vi "to string.vi"(8 "error in":errorcluster, 11 "Engine configuration in":refnum<class "Engine configuration.lvclass">) -> (0 "error out":errorcluster, 1 "data":string, 2 "version":string, 3 "Engine configuration out":refnum<class "Engine configuration.lvclass">)   [LabVIEW 2025, in "Abstract Engine.lvlib" / "Engine configuration.lvclass"]
doc: "Provides an interface for saving a module configuration to a file or other serialized data source. It is recommended that all children of this class store data in two sets--data required for its own initialization, and any data required for parent initialization--and that each implementation uses the <b>Call Parent Method</b> primitive to serialize parent information.Copyright 2017 National Instruments Corporation\n\nLicensed under the Apache License, Version 2.0 (the \"License\"); you may not use this file except in compliance with the License. You may obtain a copy of the License at http://www.apache.org/licenses/LICENSE-2.0\nUnless required by applicable law or agreed to in writing, software distributed under the License is distributed on an \"AS IS\" BASIS, WITHOUT WARRANTIES OR CONDITIONS OF ANY KIND, either express or implied. See the License for the specific language governing permissions and limitations under the License."
uses:
  Engine configuration.lvclass
  Engine configuration.lvclass/Engine configuration.ctl
  Users/Public/Documents/Sandia National Labs/TSS Plugin/CEF.lvlibp/serializable configuration/CEF_serializable configuration.lvclass
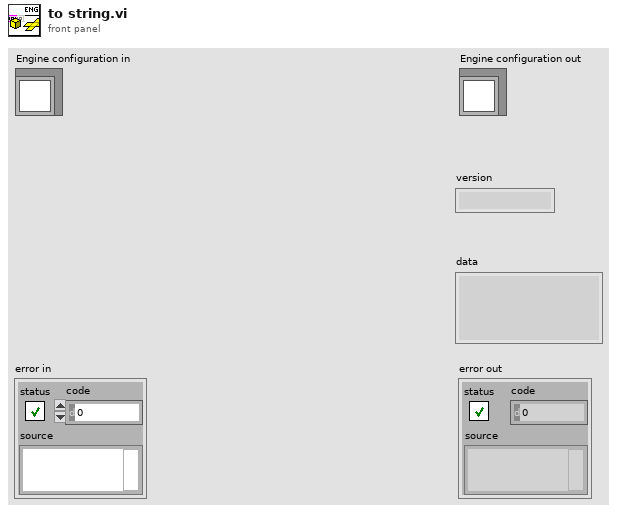
[diagram p1: front panel]
types:
  T1 = typedef "Abstract Engine.lvlib/Engine configuration.lvclass/Engine Setting.ctl" = cluster{"Enabled":bool, "IP Address":string, "Port":i32, "Initialize Order":i32, "Description":string, "Version":string, "Type":string}
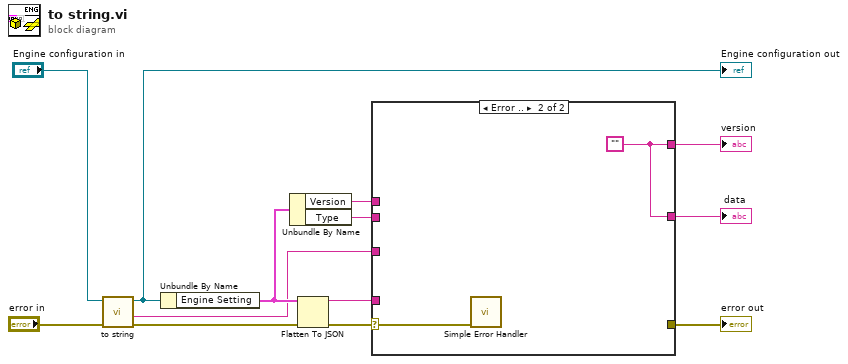
[diagram p0: block diagram]
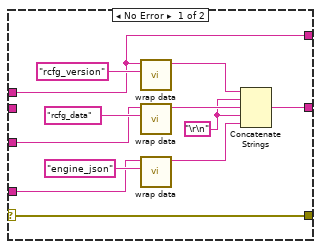
[diagram p2: hidden frame]
diagram:
  n1 = call-parent "to string.vi"("error in"="error in", "CEF_Configuration in"="Engine configuration in") -> ("error out"=w10:errorcluster, "data"=w4:string, "CEF_Configuration out"=w11:refnum<class "Engine configuration.lvclass">)  [unwired: 6 in, 1 out]
  "Engine configuration out" <- w11
  n2 = Unbundle By Name(w11) -> ("Engine Setting"=w9:T1)
  n3 = Unbundle By Name(w9) -> ("Version"=w3:string, "Type"=w1:string)
  n4 = Flatten To JSON(anything=w9, error in (no error)=w10) -> (JSON string=w7:string, 11:w8:errorcluster)  [unwired: 1 in]
  n5 = case shown="Error .." w8 {
    selector: w8 -> [w25 w26]
    tunnel: [w25 _] -> w5
    tunnel: w7 -> [w21 _]
    tunnel: w4 -> [w19 _]
    tunnel: [w18 w27] -> w6
    tunnel: w3 -> [w14 _]
    tunnel: [w14 w27] -> w2
    tunnel: w1 -> [_ _]
    frame No Error {
      w16 = "\r\n"
      n6 = call "wrap data.vi"("identifier"="rcfg_version" ("additional identifier"), "data to wrap"=w14) -> ("wrapped data"=w15:string)  [unwired: 9 in]
      n7 = call "wrap data.vi"("identifier"="rcfg_data" ("additional identifier"), "data to wrap"=w19) -> ("wrapped data"=w24:string)  [unwired: 9 in]
      n8 = call "wrap data.vi"("identifier"="engine_json" ("additional identifier"), "data to wrap"=w21) -> ("wrapped data"=w23:string)  [unwired: 9 in]
      n9 = Concatenate Strings(w15, w16, w24, w16, w23) -> (w18:string)
    }
    frame Error {
      w27 = ""
      n10 = call <vilib>:"Simple Error Handler.vi"("error in (no error)"=w26) -> ()  [unwired: 4 in, 5 out]
    }
  }
  "error out" <- w5
  "version" <- w2
  "data" <- w6
